vi "Read Part Specfic Parameters.vi"(8 "error in (no error)":errorcluster, 10 "Part name":string, 11 "PartsList":T2(array[cluster])) -> (0 "error out":errorcluster, 3 "PartSpecificParameters":T1)   [LabVIEW 2019, in "Machine Interface.lvclass"]
uses:
  Machine Interface.lvclass
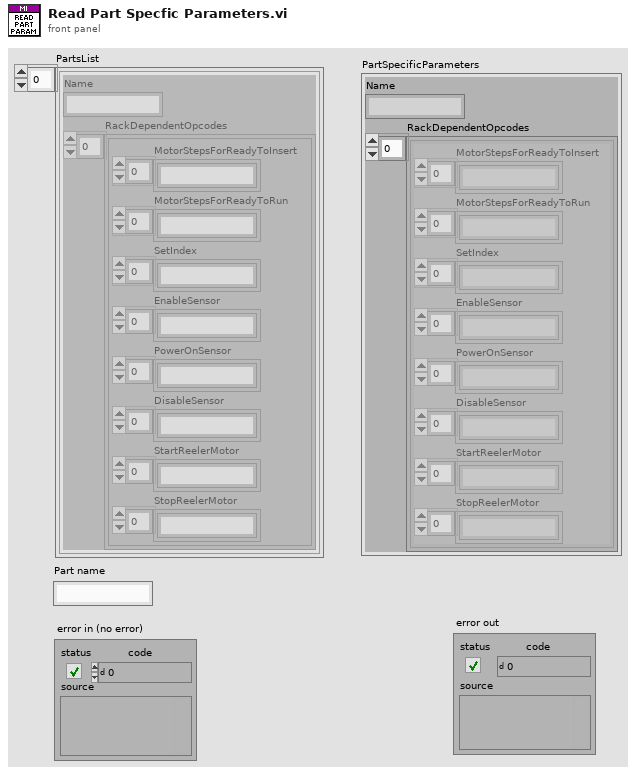
[diagram p1: front panel]
types:
  T1 = cluster{"Name":string, "RackDependentOpcodes":cluster{"MotorStepsForReadyToInsert":string[], "MotorStepsForReadyToRun":string[], "SetIndex":string[], "EnableSensor":string[], "PowerOnSensor":string[], "DisableSensor":string[], "StartReelerMotor":string[], "StopReelerMotor":string[]}[]}
  T2 = cluster{"Name":string, "RackDependentOpcodes":cluster{"MotorStepsForReadyToInsert":string[], "MotorStepsForReadyToRun":string[], "SetIndex":string[], "EnableSensor":string[], "PowerOnSensor":string[], "DisableSensor":string[], "StartReelerMotor":string[], "StopReelerMotor":string[]}[]}[]
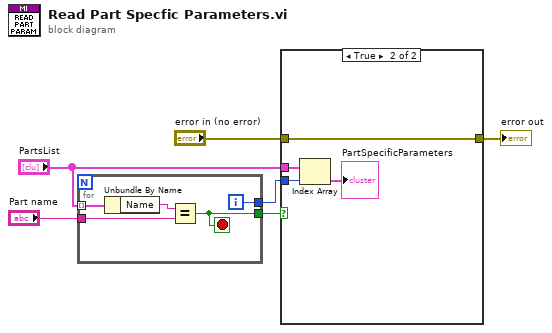
[diagram p0: block diagram]
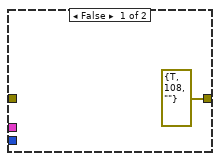
[diagram p2: hidden frame]
diagram:
  n1 = for {
    tunnel: "PartsList" -> [w11] mode=indexing
    tunnel: [w9] -> w5
    tunnel: [w8] -> w3
    tunnel: "Part name" -> [w7]
    i -> [w9]
    stop <- w8 stop-if-true
    n2 = Unbundle By Name(w11) -> ("Name"=w10:string)
    n3 = Equal?(x=w10, y=w7) -> (x = y?=w8:bool)
  }
  n4 = case shown="True" w3 {
    tunnel: "PartsList" -> [_ w16]
    tunnel: w5 -> [_ w15]
    tunnel: [errorcluster {"status"=TRUE, "code"=108, "source"=""} ("error in (no error)") w14] -> w2
    tunnel: "error in (no error)" -> [_ w14]
    frame False {
    }
    frame True {
      n5 = Index Array(array=w16, index=w15) -> (element=→"PartSpecificParameters":T1)
    }
  }
  "error out" <- w2
